vi "Get Result Sequence.vi"(8 "error in (no error)":errorcluster caption="entrée d'erreur (pas d'erreur)", 10 "Function":enum16{"Get Result", "Reset", "Set Result"}(ring), 11 "Result In":bool) -> (0 "error out":errorcluster caption="sortie d'erreur", 3 "Result Out":bool)   [LabVIEW 2020]
uses:
  TypeDef/Variable Printable.ctl
  Library Commun.lvlib
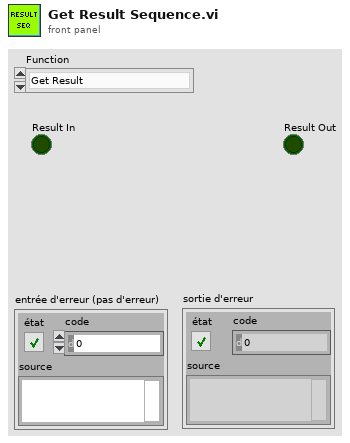
[diagram p1: front panel]
types:
  T1 = typedef "Variable Printable.ctl" = string
  T2 = enum16{"Get Variable", "Get All Variables", "Set Variable", "Delete Variable", "Delete All Variable"}
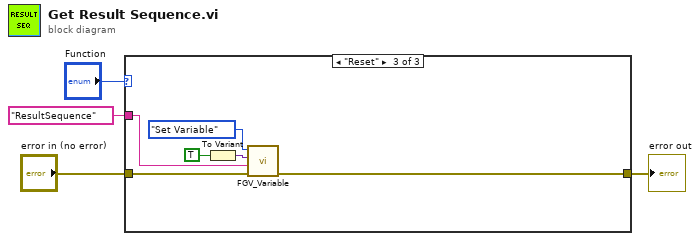
[diagram p0: block diagram]
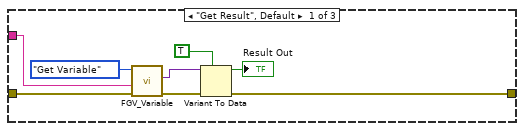
[diagram p2: hidden frame]
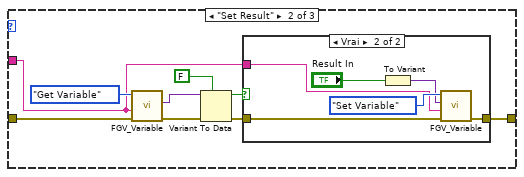
[diagram p3: hidden frame]
diagram:
  n1 = case shown="\"Reset\"" "Function" {
    tunnel: T1 "ResultSequence" ("Variable") -> [w11 w13 w34]
    tunnel: "error in (no error)" -> [w10 w15 w29]
    tunnel: [w8 w21 w33] -> w2
    frame "Get Result", Default {
      n2 = call "FGV_Variable.vi"("error in (no error)"=w10, "Variable"=w11, "Function"=T2."Get Variable") -> ("error out"=w9:errorcluster, "Data Out"=w7:variant)  [unwired: 6 in, 1 out]
      n3 = Variant To Data(error in=w9, type=TRUE, Variant=w7) -> (data=→"Result Out":bool, error out=w8:errorcluster)
    }
    frame "Set Result" {
      n4 = call "FGV_Variable.vi"("error in (no error)"=w15, "Variable"=w13, "Function"=T2."Get Variable") -> ("error out"=w20:errorcluster, "Data Out"=w19:variant)  [unwired: 6 in, 1 out]
      n5 = Variant To Data(error in=w20, type=FALSE, Variant=w19) -> (data=w14:bool, error out=w16:errorcluster)
      n6 = case shown="Vrai" w14 {
        tunnel: w13 -> [_ w27]
        tunnel: w16 -> [w22 w26]
        tunnel: [w22 w25] -> w21
        frame False {
        }
        frame True {
          n7 = To Variant(anything="Result In") -> (Variant=w23:variant)
          n8 = call "FGV_Variable.vi"("error in (no error)"=w26, "Variable"=w27, "Data In"=w23, "Function"=T2."Set Variable") -> ("error out"=w25:errorcluster)  [unwired: 5 in, 2 out]
        }
      }
    }
    frame "Reset" {
      n9 = To Variant(anything=TRUE) -> (Variant=w31:variant)
      n10 = call "FGV_Variable.vi"("error in (no error)"=w29, "Variable"=w34, "Data In"=w31, "Function"=T2."Set Variable") -> ("error out"=w33:errorcluster)  [unwired: 5 in, 2 out]
    }
  }
  "error out" <- w2
